vi "cuda_dll_test main.vi"() -> ()   [LabVIEW 2017]
panel:
  out "rdp_mean out":sgl[][](array[numeric])
  out "yc out":sgl[](array[numeric])
  out "xc out":sgl[](array[numeric])
  out "rdp_profile out":sgl[][](array[numeric])
  in  "sampling rate":i32=5
  out "y_qi_out":sgl[][](array[numeric])
  out "x_qi_out":sgl[][](array[numeric])
  out "rdp_profile":sgl[][][](array[numeric])
  out "Image":T1(plugin-control)
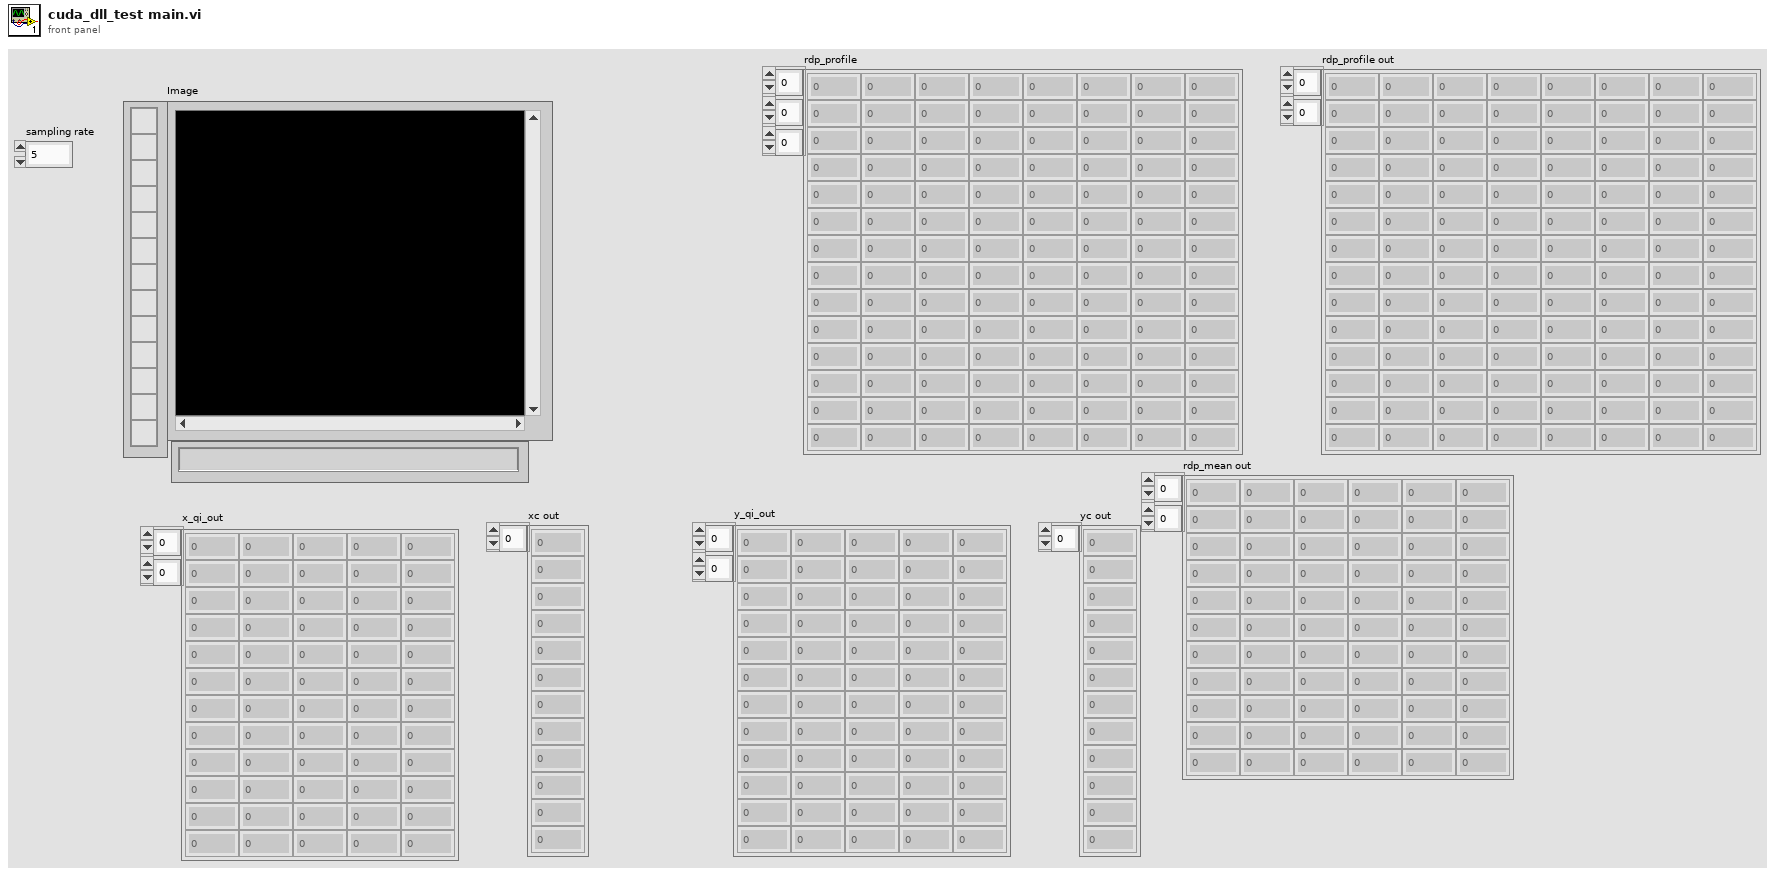
[diagram p1: front panel]
types:
  T1 = typedef "IMAQ Image.ctl" = refnum<image>
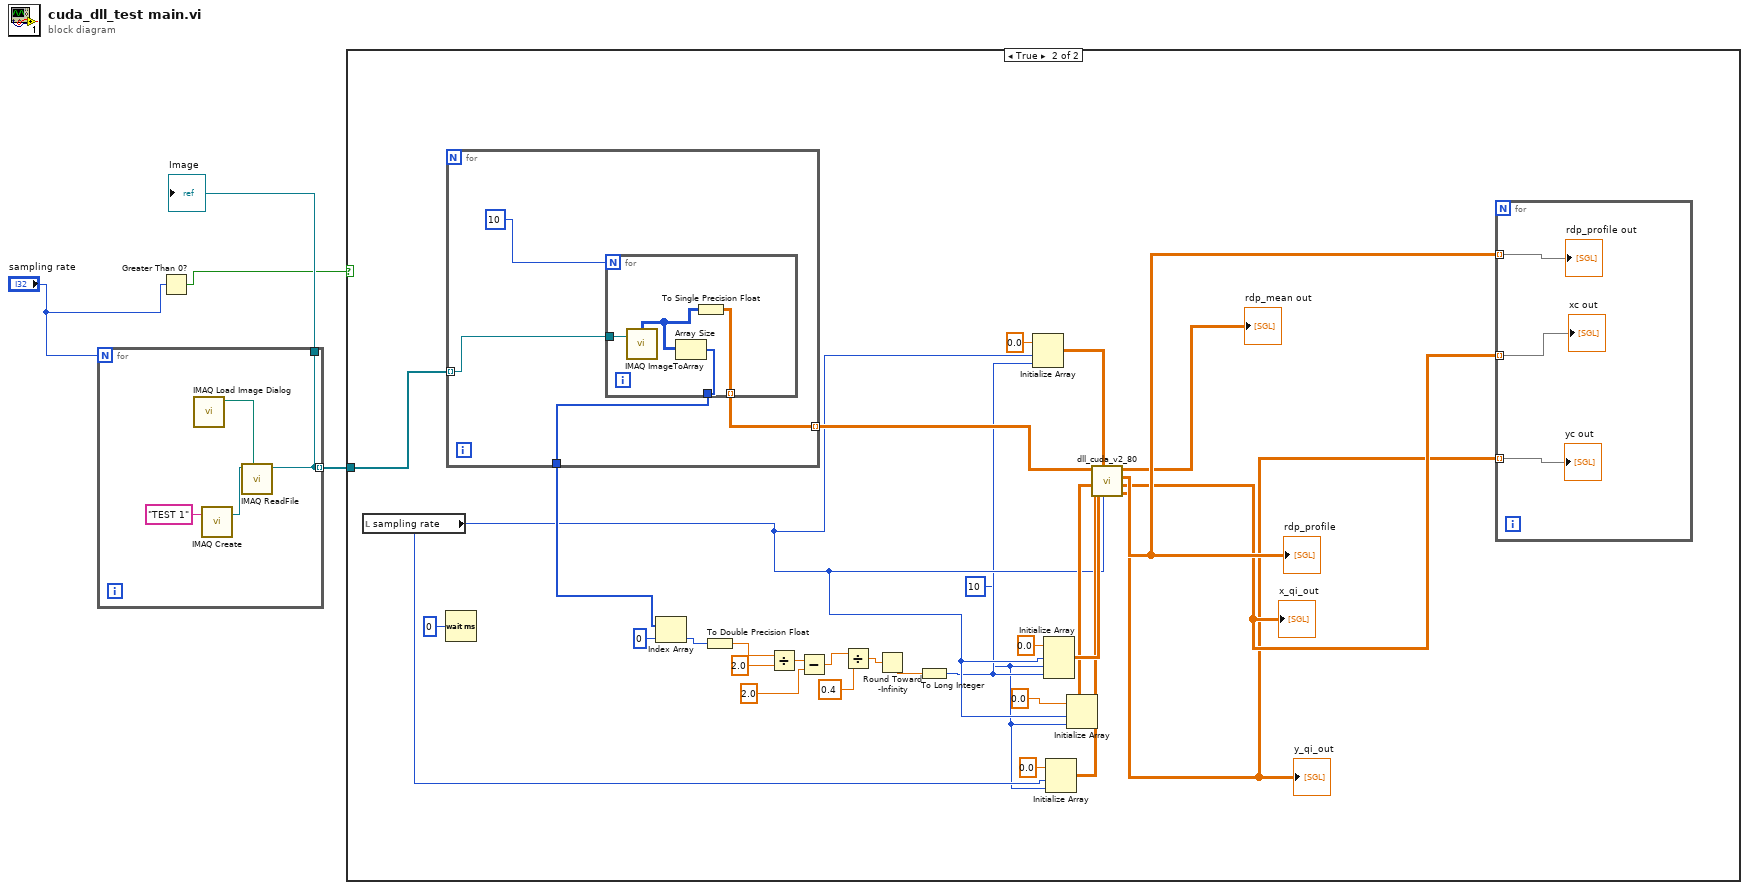
[diagram p0: block diagram]
diagram:
  n1 = for {
    N: "sampling rate" -> [_]
    tunnel: [w6] -> w4
    tunnel: [w6] -> w3 mode=indexing
    n2 = call "IMAQ Load Image Dialog"() -> ("Path"=w5:path)  [unwired: 9 in, 2 out]
    n3 = call "IMAQ Create"("Image Name"="TEST 1") -> ("New Image"=w8:T1)  [unwired: 4 in, 1 out]
    n4 = call "IMAQ ReadFile"("File Path"=w5, "Image"=w8) -> ("Image Out"=w6:T1)  [unwired: 5 in, 4 out]
  }
  "Image" <- w4
  n5 = Greater Than 0?(x="sampling rate") -> (x > 0?=w1:bool)
  n6 = case shown="True" w1 {
    tunnel: w3 -> [_ w37]
    frame False {
    }
    frame True {
      w13 = 10 ("n_frame")
      n7 = local read "sampling rate"() -> (w15:i32)
      n8 = Wait (ms)(milliseconds to wait=u32 0) -> ()  [unwired: 1 out]
      n9 = for {
        tunnel: w37 -> [w42] mode=indexing
        tunnel: [w43] -> w22
        tunnel: [w41] -> w20 mode=indexing
        n10 = for {
          N: 10 -> [_]
          tunnel: w42 -> [w48]
          tunnel: [w46] -> w43
          tunnel: [w45] -> w41 mode=indexing
          n11 = call "IMAQ ImageToArray"("Image"=w48) -> ("Image Pixels (U8)"=w47:u8[][])  [unwired: 3 in, 4 out]
          n12 = Array Size(array=w47) -> (size(s)=w46:i32[])
          n13 = To Single Precision Float(number=w47) -> (single precision float=w45:sgl[][])
        }
      }
      n14 = Index Array(array=w22, index=0) -> (element=w9:i32)
      n15 = To Double Precision Float(number=w9) -> (double precision float=w36:dbl)
      n16 = Divide(x=w36, y=2.0) -> (x/y=w35:dbl)
      n17 = Subtract(x=w35, y=2.0) -> (x-y=w34:dbl)
      n18 = Divide(x=w34, y=0.4) -> (x/y=w33:dbl)
      n19 = Round Toward -Infinity(1:w33) -> (0:w32:dbl)
      n20 = To Long Integer(number=w32) -> (32bit integer=w14:i32)
      n21 = Initialize Array(sgl 0.0 ("element"), w15, w14) -> (w11:sgl[][])
      n22 = Initialize Array(sgl 0.0 ("element"), w15, w13, w14) -> (w27:sgl[][][])
      n23 = Initialize Array(sgl 0.0 ("element"), w15, w13) -> (w23:sgl[][])
      n24 = Initialize Array(sgl 0.0 ("element"), w15, w13) -> (w24:sgl[][])
      n25 = call "dll_cuda_v2_80.vi"("n_stream"=w15, "rdp_mean"=w11, "yc"=w23, "xc"=w24, "rdp_profile"=w27, "img_mat 4d"=w20) -> ("yc out"=w16:sgl[][], "xc out"=w17:sgl[][], "rdp_profile out"=w18:sgl[][][], "rdp_mean out"=→"rdp_mean out":sgl[][])  [unwired: 2 in]
      "rdp_profile" <- w18
      "y_qi_out" <- w16
      "x_qi_out" <- w17
      n26 = for {
        tunnel: w18 -> [w40] mode=indexing
        tunnel: w17 -> [w39] mode=indexing
        tunnel: w16 -> [w38] mode=indexing
        "rdp_profile out" <- w40
        "xc out" <- w39
        "yc out" <- w38
      }
    }
  }
